vi "remote.Close Property.vi"(0 "SLSC Remote in":refnum<class "SLSC Remote.lvclass">, 5 "property":refnum<k21>, 11 "error in (no error)":errorcluster) -> (4 "SLSC Remote out":refnum<class "SLSC Remote.lvclass">, 15 "error out":errorcluster)   [LabVIEW 2016, in "SLSC Interfaces.lvlib" / "SLSC Remote.lvclass"]
uses:
  SLSC Remote.lvclass
  <vilib>/NI/NI JSONRPC Server Framework/Classes/Server/JSONRPC Server.lvclass
  <vilib>/httpClient/LabVIEWHTTPClient.lvlib
  <vilib>/httpClient/POSTBuffer.vi
  <vilib>/NI/JSON Support for LabVIEW/JSON Data Classes/JSON Helper/JSON Helper.lvclass
  <vilib>/NI/JSON Support for LabVIEW/JSON Data Classes/JSON Object/New JSON Object (Single String).vi
  <vilib>/NI/JSON Support for LabVIEW/JSON Data Classes/JSON Object/JSON Object.lvclass
  <vilib>/NI/NI JSONRPC Server Framework/Classes/Server/Format Client Request (Auto-Increment).vi
  <vilib>/NI/NI JSONRPC Server Framework/Classes/Server/Parse Response (Object).vi
  C:/Program Files (x86)/National Instruments/LabVIEW 2016/vi.lib/NI/JSON Support for LabVIEW/JSON Data Classes/JSON Structured Type/JSON Structure.lvclass
  C:/Program Files (x86)/National Instruments/LabVIEW 2016/vi.lib/NI/JSON Support for LabVIEW/JSON Data Classes/JSON Datatype/JSON Null.lvclass
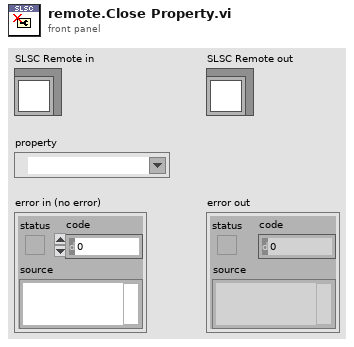
[diagram p1: front panel]
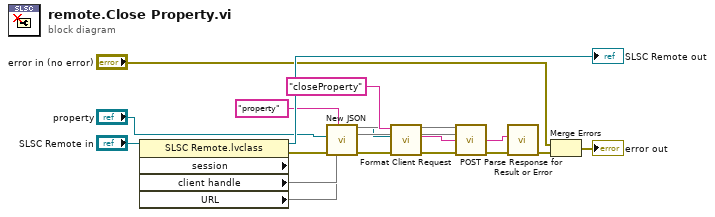
[diagram p0: block diagram]
diagram:
  n1 = property class="SLSC Remote.lvclass" props=["session", "client handle", "URL"](reference="SLSC Remote in") -> (reference out=→"SLSC Remote out":refnum<class "SLSC Remote.lvclass">, error out=w15:errorcluster, "client handle"=w11, "URL"=w10)  [unwired: 1 in, 1 out]
  n2 = call-poly <vilib>:"New JSON.vi"("key"="property" ("Name"), "error in (no error)"=w15, "value"="property") -> ("error out"=w14:errorcluster, "JSON Object out"=w1:refnum<class "JSON Object.lvclass">)  [unwired: 7 in]
  n3 = call-poly <vilib>:"Format Client Request.vi"("error in (no error)"=w14, "JSON in"=w1, "method"="closeProperty") -> ("error out"=w9:errorcluster, "Request String"=w12:string)  [unwired: 7 in]
  n4 = call-poly <vilib>:"POST.vi"("client handle"=w11, "url"=w10, "buffer"=w12, "error in (no error)"=w9) -> ("body"=w8:string, "error out"=w7:errorcluster)  [unwired: 8 in, 2 out]
  n5 = call-poly <vilib>:"Parse Response for Result or Error.vi"("error in"=w7, "Response String In"=w8) -> ("error out"=w6:errorcluster)  [unwired: 7 in, 2 out]
  n6 = Merge Errors("error in (no error)", w6) -> (→"error out":errorcluster)
